vi "MiC.vi"() -> ()   [LabVIEW 2018]
uses:
  <vilib>/DAQmx/read.llb/DAQmx Read (Analog Wfm 1Chan NSamp).vi
  <vilib>/DAQmx/create/channels.llb/DAQmx Create Channel (AI-Voltage-Basic).vi
  <vilib>/DAQmx/configure/timing.llb/DAQmx Timing (Sample Clock).vi
  <vilib>/DAQmx/miscellaneous.llb/DAQmx Fill In Error Info.vi
panel:
  out "웨이브폼 차트":waveform(dbl)(graph)
  in  "정지":bool
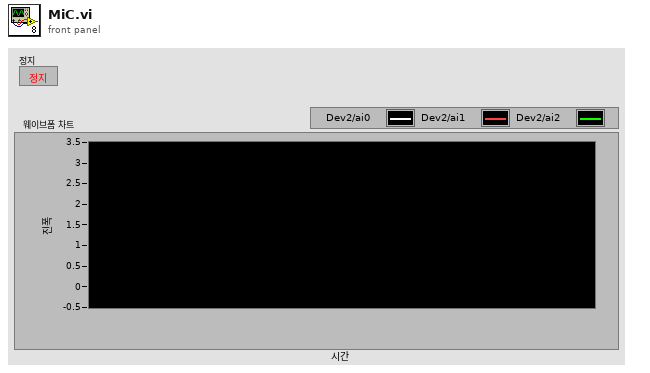
[diagram p1: front panel]
types:
  T1 = enum16{"open", "open or create", "create or replace", "create", "open (read-only)"}
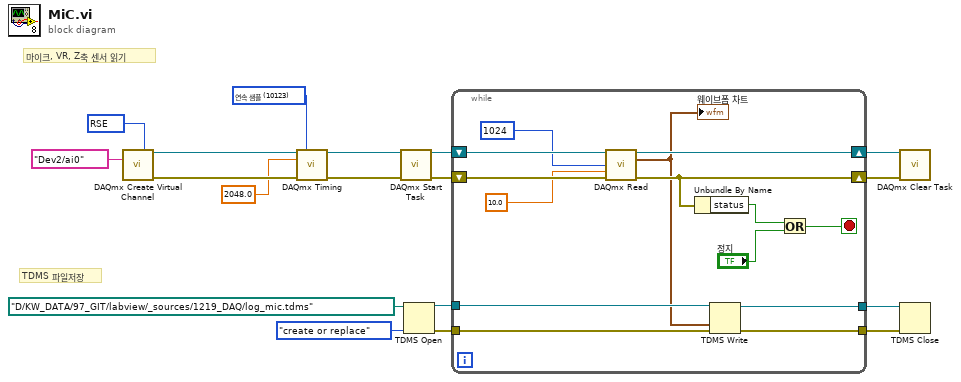
[diagram p0: block diagram]
diagram:
  w7 = 10123 items=["유한 샘플"=10178, "연속 샘플"=10123, "하드웨어 타이밍에 의한 단일 포인트"=12522] ("sample mode")
  w8 = 10083 items=["기본"=-1, "RSE"=10083, "NRSE"=10078, "차동"=10106, "유사 차동"=12529] ("input terminal configuration")
  # "마이크, VR, Z축 센서 읽기"
  # "TDMS 파일저장"
  n1 = call-poly <vilib>:"DAQmx Create Virtual Channel.vi"("input terminal configuration"=w8, "physical channels"=tag "Dev2/ai0") -> ("task out"=w18:refnum<k21>, "error out"=w17:errorcluster)  [unwired: 12 in]
  n2 = call-poly <vilib>:"DAQmx Timing.vi"("task/channels in"=w18, "sample mode"=w7, "rate"=2048.0, "error in"=w17) -> ("task out"=w16:refnum<k21>, "error out"=w15:errorcluster)  [unwired: 10 in]
  n3 = call <vilib>:"DAQmx Start Task.vi"("task/channels in"=w16, "error in"=w15) -> ("task out"=w14:refnum<k21>, "error out"=w13:errorcluster)  [unwired: 12 in]
  n4 = TDMS Open(10:T1."create or replace" ("동작(0:open)"), 11:path "D:/KW_DATA/97_GIT/labview/_sources/1219_DAQ/log_mic.tdms" ("파일 경로")) -> (0:w5:errorcluster, 3:w6:refnum<k34>)  [unwired: 5 in]
  n5 = while {
    shift-right: [w30] -> w12
    shift-left: w14 -> [w32]
    shift-right: [w27] -> w11
    shift-left: w13 -> [w31]
    tunnel: w6 -> [w23]
    tunnel: w5 -> [w22]
    tunnel: [w21] -> w4
    tunnel: [w20] -> w3
    stop <- w24 stop-if-true
    n6 = call-poly <vilib>:"DAQmx Read.vi"("task/channels in"=w32, "number of samples per channel"=1024, "timeout"=10.0, "error in"=w31) -> ("task out"=w30:refnum<k21>, "data"=w19:waveform(dbl), "error out"=w27:errorcluster)  [unwired: 9 in]
    "웨이브폼 차트" <- w19
    n7 = Unbundle By Name(w27) -> ("status"=w26:bool)
    n8 = TDMS Write(0:w23, 9:w19, 11:w22) -> (4:w21:refnum<k34>, 15:w20:errorcluster)  [unwired: 3 in, 2 out]
    n9 = Or(x=w26, y="정지") -> (x .or. y?=w24:bool)
  }
  n10 = call <vilib>:"DAQmx Clear Task.vi"("task in"=w12, "error in"=w11) -> ()  [unwired: 13 in, 1 out]
  n11 = TDMS Close(8:w3, 11:w4) -> ()  [unwired: 2 out]
